vi "Read Root.vi"(11 "Spawn in":refnum<class "Spawn.lvclass">) -> (2 "Root":bool)   [LabVIEW 2025, in "jettl.lvlib" / "Spawn.lvlib" / "Spawn.lvclass"]
uses:
  Spawn.lvclass
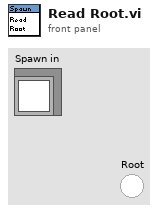
[diagram p1: front panel]
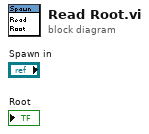
[diagram p0: block diagram]
diagram:
